vi "MFLI controller -- V1.vi"(6 "pm lorentzian":T1={"Amplitude"=0.011556077084443558, "omega(0)"=1994480.3546612726, "Gamma"=468.65303298958196, "phase"=4.673413347310273, "Q"=4255.771784806969, "Norm  Ampl"=nan, "z (inf)"=2.6527949823343002e-05+0.0007477540585896028i, "4corners"={"z (-pi/2)"=9.277908004825974e-07+0.0007240755403629966i, "z(inf)"=2.6527949823343002e-05+0.0007477540585896028i, "z (pi/2)"=2.8494315967368497e-06+0.0007733542176124632i, "z center"=1.8886111986097237e-06+0.0007487148789877299i, "z(0)"=-2.2750727426123552e-05+0.000749675699385857i, "radius"=2.4658065287076567e-05}} {"z (inf)" format="%#9_9f"; "Q" format="%#9_9f"; "phase" format="%#9_9f"; "Gamma" format="%#9_9f"; "omega(0)" format="%#9_9f"}, 7 "MFLI controller action":T3, 8 "Error In":errorcluster, 9 "sweep parameters":T4={"scan type"=enum."linear", "N"=200, "cursor window"={"left"=2378.60310421286, "right "=2421.6740576496672, "center"=2421.6740576496672, "window"=2421.6740576496672, "cursors"=[], "relative"=0, "absolute"=0, "fixed vertical offset"=2421.6740576496672, "vertical offset"=2421.6740576496672, "skew"=2421.6740576496672, "default window frac"=2421.6740576496672, "kind"=enum."skewed", "skew.left"=2421.6740576496672, "skew.right"=2421.6740576496672, "Plot ref"=refnum, "wing order"=enum."back"}}, 10 "Address":string="DEV3523") -> (0 "Error Out":errorcluster, 1 "Voltage out (V)":cdb[](array[numeric])=[1.7947140397689774e-05+0.0007833320820365352i, 2.4161799481718794e-05+0.000775952788866728i, 1.1398171168621245e-05+0.000786642257900688i, 2.1378172412082557e-05+0.0007803848389655606i, 2.3527732690994892e-05+0.0007832482826747523i, 2.018710709966375e-05+0.000775222845149317i, 2.1052965461761493e-05+0.0007926707916558383i, 2.578223850561299e-05+0.0007823212803731786i, 3.539618410572311e-05+0.000787718994219253i, 2.597151232578711e-05+0.0007817704065018801i, 1.8686171805884874e-05+0.0007845914493356854i, 1.9525315696386483e-05+0.0007805387882637953i, 2.4826921249368033e-05+0.0007881234674194581i, 2.272879706177131e-05+0.0007813422850312608i, 3.06221404697413e-05+0.0007823486263319492i, 2.258400939616162e-05+0.0007913708833571255i, 2.631790122834116e-05+0.0007837787712575242i, 1.877589665213771e-05+0.0007839841799029761i, 2.6429055493472353e-05+0.0007841953035371732i, 2.531443173334934e-05+0.0007816207088595043i, 1.874285359377707e-05+0.0007808713190342089i, 1.3108402421252441e-05+0.0007954138097471226i, 3.648735100939127e-05+0.0007923069644049057i, 1.780208141322794e-05+0.000787914506584111i, 1.0674633557646736e-05+0.0007985997639146586i, 1.546188714204973e-05+0.0007832137363310591i, 2.7415050861775486e-05+0.0007861266083720606i, 1.892095325137887e-05+0.00078571478332542i, 1.7149941209119945e-05+0.0007909710678965998i, 2.3090619534723823e-05+0.0007954700335726445i, 1.4252127066260151e-05+0.0007941394739956062i, 2.5280803103312197e-05+0.0007950770857587566i, 3.212975080358819e-05+0.0007937076512587993i, 1.760575986225483e-05+0.0007908437662837823i, 1.5797629612106515e-05+0.0008016906241041951i, 2.0336565623666577e-05+0.0007986538499861476i, 1.485039288721422e-05+0.000805913067569182i, 2.800021108771304e-05+0.0008038452672883727i, 3.085236077699336e-05+0.0008007500940235448i, 2.129881492750763e-05+0.0008020268042622464i, 3.554295448602157e-06+0.0008061419277043423i, 2.6006880974309018e-05+0.0008047380041059882i, 2.6980288340482813e-05+0.0007933068495095234i, 1.1121641205596253e-05+0.0007879329640180243i, 1.4052702939489842e-05+0.0007929102356114531i, 2.1013801330835356e-05+0.000794124604529898i, 1.626598558143133e-05+0.0007992144555578133i, 1.9885387417361182e-05+0.0008023925593677921i, 2.3694890148735325e-05+0.0007999127658822845i, 8.742127167842653e-06+0.0007970248265530325i, 1.2390541039186939e-05+0.000802933229265029i, 1.483243933116921e-05+0.0007945130842291504i, 9.538450384118407e-06+0.0008015181142112527i, 8.452853567039068e-06+0.0007996583290257916i, 9.257628812788116e-06+0.0008072990894900408i, 1.1681645701650892e-05+0.0008048214754999279i, 6.991344778460933e-06+0.0008067030961880879i, 6.70006580337213e-06+0.0008073005909864577i, 1.3001539764426547e-06+0.0008096541275858048i, 9.044858780017961e-06+0.0008092305338603379i, 6.8739954989232195e-06+0.0008196877992760521i, 1.1866893865625335e-05+0.0008081127484902058i, 1.4235732848233533e-05+0.0008109049546023166i, -7.253909274414909e-07+0.0008132737160652528i, 1.1919072953182212e-06+0.0008099574513290134i, 6.0822942440166985e-06+0.0008105701149382865i, 6.107721292751761e-07+0.0008081147192787912i, -6.260924016914232e-07+0.0008023573773627882i, 1.0163690665722533e-05+0.0008194391328646849i, 4.480674014968536e-06+0.0008205849743930445i, 4.8973529856892366e-06+0.0008076386787247464i, 5.6581191210095015e-06+0.000806127479826389i, -4.4087822711164575e-06+0.0008059624845711934i, 1.4510394587162305e-06+0.0008098497735230208i, -1.1778062880821662e-05+0.000813252261005252i, -1.4585081809649263e-06+0.0008067446723734249i, -2.049438852028277e-06+0.0008100198027864578i, -1.0382074911664064e-05+0.0008125615988908855i, -9.025509273571018e-06+0.000799131903666445i, -2.9031801738195978e-05+0.0008013498166180281i, -1.503670128178013e-05+0.0008049771236715908i, -9.824583841899107e-06+0.0008017113021785598i, -1.8305930062549926e-05+0.000801634818288597i, -8.343519821590533e-06+0.0007944148238707005i, -1.7342980100134644e-05+0.0008019266261863711i, -2.5805486655258495e-05+0.0008042511662542381i, -1.4609085477944594e-05+0.0007968365461772709i, -3.225810668394559e-05+0.0008040385739204086i, -1.5925020670699562e-05+0.0007896679550539058i, -2.9721156155325662e-05+0.0007966369425626446i, -2.5980589283078102e-05+0.0007989693669774635i, -3.771207357449536e-05+0.0008006076206182981i, -2.389227491182575e-05+0.0007991962903134331i, -2.6431435943709224e-05+0.0007911297387391672i, -2.5510202298345777e-05+0.0007948988799588347i, -2.762797414497422e-05+0.0007836354618324298i, -2.673361597360269e-05+0.0007763990308588398i, -3.259733873185462e-05+0.000779768005990542i, -3.222723298379179e-05+0.0007828007824787327i, -2.828513404599954e-05+0.0007775276290306113i, -2.7442523833547298e-05+0.000793928944281358i, -3.3840638588211066e-05+0.0007739791457684968i, -3.521552033589221e-05+0.0007752803450679017i, -3.060214993523709e-05+0.0007727985724455364i, -3.3001774961139156e-05+0.0007626825050958754i, -2.7123296631466546e-05+0.0007718388371642902i, -4.255257124748806e-05+0.0007669934247440899i, -3.38616905459171e-05+0.0007702236915413861i, -1.6438046456581025e-05+0.0007687605220429108i, -2.1381155726845848e-05+0.0007643824005910026i, -2.3810201257203493e-05+0.0007613015392465492i, -1.9462442471918776e-05+0.0007633144454623645i, -1.3585483527818204e-05+0.0007618983596237723i, -1.0020322802721557e-05+0.0007542783314976581i, -1.6568035020492665e-05+0.0007604883692166231i, -2.298965314341451e-05+0.0007605745114614172i, -1.426624995789593e-05+0.0007620358437436652i, -2.0535935486666456e-05+0.0007556581560188897i, -1.7212791773991207e-05+0.0007694160367379733i, -1.3989350285665814e-05+0.0007610824084265354i, -1.400786973531673e-05+0.0007577904317961574i, -1.8543965545354192e-05+0.0007530162033055729i, -9.895804742435434e-06+0.0007541670555862725i, -1.182271182669738e-05+0.0007564713874682483i, -1.3404755357029001e-06+0.0007534417952496631i, -2.540462766068613e-07+0.0007474275871299063i, -1.3033629927126234e-05+0.0007444921079673166i, -3.0160083868227686e-06+0.0007582129479981829i, -4.11029992957941e-06+0.0007583807524470322i, 7.493713398352082e-07+0.0007579380829191913i, 2.5281812647964257e-06+0.0007541958762077274i, 8.73539368986802e-06+0.0007522473143012331i, 1.9213280530955755e-06+0.0007605324767174049i, 1.203060825731675e-05+0.0007498036420013713i, 1.0818751572551014e-05+0.0007547940269417837i, -4.571233688458752e-07+0.0007544590167344752i, 9.230090843752823e-06+0.0007623847234129125i, 7.672275192460286e-06+0.0007716896457850033i, 3.724034311421603e-06+0.0007561014117147125i, 9.7155864125662e-06+0.0007589951489191279i, 1.9036995429984916e-05+0.0007591741692719116i, 2.993680932359062e-06+0.0007534712712104994i, 1.3241246094315913e-05+0.0007587625553173011i, -2.3831181061984005e-06+0.0007575792067900815i, 1.2540396106127523e-05+0.0007558400475810648i, 1.543095500398932e-05+0.000755777378292965i, 1.1838465016666725e-05+0.0007658480220963351i, 9.470274217777834e-06+0.0007540965860302497i, 1.1865047704820388e-06+0.0007644510764610753i, 8.466614501436925e-06+0.0007562911083152517i, 1.9635644675163006e-05+0.0007559176668360705i, 1.5652852679989877e-05+0.0007649946688499482i, 1.6426636753466735e-05+0.0007582663668041872i, 1.783993128756037e-05+0.0007500404991851605i, 1.0973498727102639e-05+0.0007677684950478176i, 6.5668631545965845e-06+0.0007641153292205771i, 1.3746500234922546e-05+0.0007664765390748459i, 1.313554086582413e-05+0.0007479720215016787i, 1.625381320400517e-05+0.0007647049671020328i, 2.2693736106716893e-05+0.0007611466185671932i, 1.063844260429601e-05+0.0007676103000567756i, 8.724583869754299e-06+0.000760347093192157i, 2.9722842506345163e-05+0.0007540097204672849i, 1.6862222772198565e-05+0.000766293135282761i, 1.3051362850258507e-05+0.0007733673736354523i, 2.2415757122129878e-05+0.0007654096173430668i, 1.9622996446211543e-05+0.0007736139273376037i, 1.683381240870021e-05+0.000769355971514549i, 2.4967869902296118e-05+0.0007724409640612171i, 2.8596211545327962e-05+0.0007752939199550868i, 2.225968676640701e-05+0.0007710920251662428i, 2.1970411972993085e-05+0.0007627460700343397i, 2.5802859334681428e-05+0.0007671525469896707i, 2.615942835909015e-05+0.0007751067057729683i, 1.8932634273345313e-05+0.0007677137578110834i, 2.1265462386763993e-05+0.0007613570302130178i, 2.3909834310153683e-05+0.0007645137904720627i, 2.132736423011049e-05+0.0007730512507980843i, 2.1087956052805902e-05+0.0007702563958984105i, 2.764070526034425e-05+0.0007666090142313147i, 2.8825530239163648e-05+0.0007725496436598947i, 1.729867104820557e-05+0.0007754645204788762i, 2.487072463451332e-05+0.0007644461527692902i, 3.0526769806143105e-05+0.0007779116078184439i, 2.287845117386975e-05+0.0007798770845173779i, 2.062062215054171e-05+0.0007695059261644529i, 3.166101379526004e-05+0.0007710586797811611i, 3.2229803655377746e-05+0.0007608600021022252i, 1.7318390860162808e-05+0.000778979904629944i, 2.77694380055688e-05+0.0007824131662293659i, 1.618981594429285e-05+0.0007837812626205225i, 1.969374805457943e-05+0.0007784960435336005i, 2.6395515116600305e-05+0.0007839889300699569i, 1.9374879828210753e-05+0.0007738837953792744i, 2.6467750332230046e-05+0.0007704428527729637i, 2.345675627557808e-05+0.0007902514134248894i, 1.947387304571401e-05+0.0007802039945152633i, 2.3576121662894066e-05+0.000779339309085434i, 1.2183886115930586e-05+0.0007743616063633677i, 2.839087087866531e-05+0.0007817038850823851i], 2 "sweep time":dbl=5.15086802226142, 3 "Freq out (Hz)":dbl[](array[numeric])=[1966839.6309110236, 1980604.250263973, 1985224.7472832582, 1987541.939474813, 1988935.024090971, 1989865.2790140666, 1990530.774699402, 1991030.6713716055, 1991420.1075499407, 1991732.1886906968, 1991987.9930281865, 1992201.5787029702, 1992382.681702111, 1992538.2583730097, 1992673.4113469622, 1992791.9684604905, 1992896.857472874, 1992990.3559479269, 1993074.26226771, 1993150.01536806, 1993218.7802804522, 1993281.510355006, 1993338.993258559, 1993391.8854780952, 1993440.7385467284, 1993486.019219916, 1993528.1251697806, 1993567.3973176058, 1993604.1296157013, 1993638.5768735865, 1993670.9610699513, 1993701.47648153, 1993730.2938797704, 1993757.5639871648, 1993783.4203412689, 1993807.9816815516, 1993831.3539493254, 1993853.6319720135, 1993874.9008884, 1993895.237360179, 1993914.7106062812, 1993933.3832895095, 1993951.3122795206, 1993968.5493118234, 1993985.1415589666, 1994001.1321272748, 1994016.5604902243, 1994031.4628676944, 1994045.8725588291, 1994059.8202350016, 1994073.3341983613, 1994086.4406105939, 1994099.1636958327, 1994111.5259210719, 1994123.5481569448, 1994135.2498213276, 1994146.6490078745, 1994157.7626013076, 1994168.606381035, 1994179.1951144587, 1994189.5426411608, 1994199.6619489975, 1994209.5652430046, 1994219.2640079013, 1994228.769064887, 1994238.0906233364, 1994247.238327932, 1994256.2213017046, 1994265.0481854002, 1994273.7271735466, 1994282.2660475457, 1994290.6722060877, 1994298.9526931448, 1994307.1142237792, 1994315.163207975, 1994323.1057726797, 1994330.9477822206, 1994338.6948572523, 1994346.3523923666, 1994353.925572489, 1994361.419388173, 1994368.8386498927, 1994376.1880014255, 1994383.4719324044, 1994390.694790122, 1994397.8607906487, 1994404.974029333, 1994412.0384907408, 1994419.058058085, 1994426.036522199, 1994432.9775900966, 1994439.8848931633, 1994446.761995016, 1994453.61239907, 1994460.439555851, 1994467.246870078, 1994474.0377075572, 1994480.8154019113, 1994487.583261174, 1994494.3445742792, 1994501.1026174715, 1994507.8606606638, 1994514.621973769, 1994521.3898330317, 1994528.1675273858, 1994534.958364865, 1994541.765679092, 1994548.592835873, 1994555.443239927, 1994562.3203417796, 1994569.2276448463, 1994576.168712744, 1994583.147176858, 1994590.1667442021, 1994597.2312056099, 1994604.3444442942, 1994611.5104448209, 1994618.7333025385, 1994626.0172335175, 1994633.3665850502, 1994640.78584677, 1994648.279662454, 1994655.8528425763, 1994663.5103776907, 1994671.2574527224, 1994679.0994622633, 1994687.042026968, 1994695.0910111638, 1994703.2525417982, 1994711.5330288552, 1994719.9391873972, 1994728.4780613964, 1994737.1570495428, 1994745.9839332383, 1994754.9669070109, 1994764.1146116066, 1994773.436170056, 1994782.9412270417, 1994792.6399919384, 1994802.5432859454, 1994812.6625937822, 1994823.0101204843, 1994833.598853908, 1994844.4426336354, 1994855.5562270684, 1994866.9554136153, 1994878.6570779982, 1994890.679313871, 1994903.0415391102, 1994915.764624349, 1994928.8710365817, 1994942.3849999413, 1994956.3326761138, 1994970.7423672485, 1994985.6447447187, 1995001.0731076682, 1995017.0636759764, 1995033.6559231195, 1995050.8929554224, 1995068.8219454335, 1995087.4946286618, 1995106.967874764, 1995127.304346543, 1995148.5732629295, 1995170.8512856176, 1995194.2235533914, 1995218.784893674, 1995244.6412477782, 1995271.9113551725, 1995300.728753413, 1995331.2441649917, 1995363.6283613564, 1995398.0756192417, 1995434.8079173372, 1995474.0800651624, 1995516.1860150269, 1995561.4666882146, 1995610.3197568478, 1995663.211976384, 1995720.694879937, 1995783.4249544907, 1995852.189866883, 1995927.942967233, 1996011.849287016, 1996105.347762069, 1996210.2367744525, 1996328.7938879807, 1996463.9468619332, 1996619.523532832, 1996800.6265319728, 1997014.2122067565, 1997270.016544246, 1997582.0976850023, 1997971.5338633375, 1998471.430535541, 1999136.9262208764, 2000067.1811439719, 2001460.26576013, 2003777.4579516847, 2008397.95497097])   [LabVIEW 2016]
uses:
  <instrlib>/Zurich Instruments LabOne/Zurich Instruments LabOne.lvlib
  MFLI controller action.ctl
  cursor winow.ctl
  sweep parameters.ctl
  circle corners.ctl
  lorentzian.ctl
panel:
  out "Thermometer":i32(slide) scale=0.0..100.0
  out "Selected Device":string="DEV3523"
  out "ind":i64=-1
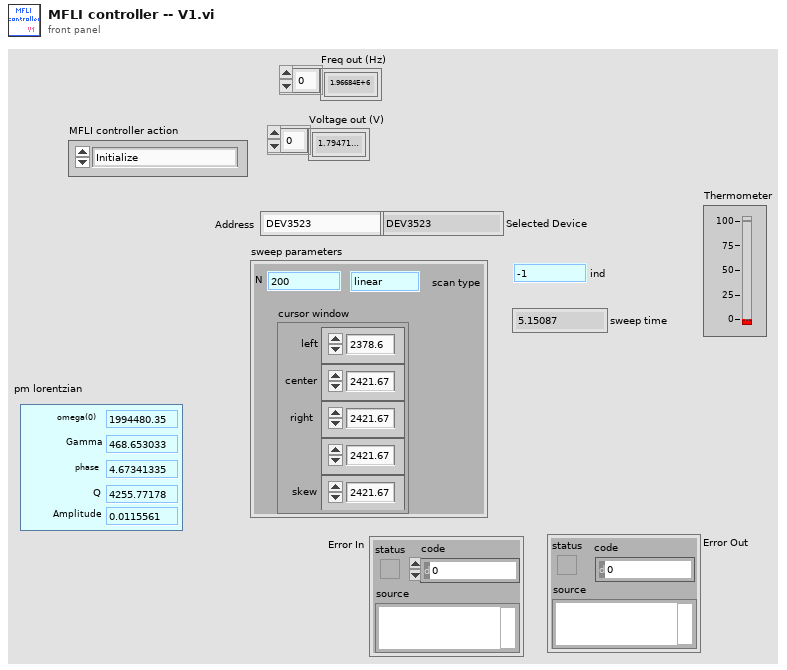
[diagram p1: front panel]
types:
  T1 = typedef "lorentzian.ctl" = cluster{"Amplitude":dbl, "omega(0)":dbl, "Gamma":dbl, "phase":dbl, "Q":dbl, "Norm  Ampl":dbl, "z (inf)":cdb, "4corners":T2}
  T2 = typedef "circle corners.ctl" = cluster{"z (-pi/2)":cdb, "z(inf)":cdb, "z (pi/2)":cdb, "z center":cdb, "z(0)":cdb, "radius":dbl}
  T3 = typedef "MFLI controller action.ctl" = enum16{"Initialize", "Scan frequency", "open", "close", "read", "circle PLL"}
  T4 = typedef "sweep parameters.ctl" = cluster{"scan type":enum16{"linear", "arctan"}, "N":i64, "cursor window":T5}
  T5 = typedef "cursor winow.ctl" = cluster{"left":dbl, "right ":dbl, "center":dbl, "window":dbl, "cursors":i32[], "relative":i32, "absolute":i32, "fixed vertical offset":dbl, "vertical offset":dbl, "skew":dbl, "default window frac":dbl, "kind":enum16{"symmetric", "skewed", "fancy"}, "skew.left":dbl, "skew.right":dbl, "Plot ref":refnum<vi>, "wing order":enum16{"forw", "back"}}
  T6 = typedef "Zurich Instruments LabOne.lvlib/ziTypeHandle.ctl" = cluster{"handleValid":bool, "Conn":u64, "Path Prefix":string, "Handle":u64, "Connected":bool, "Clockbase(s)":dbl}
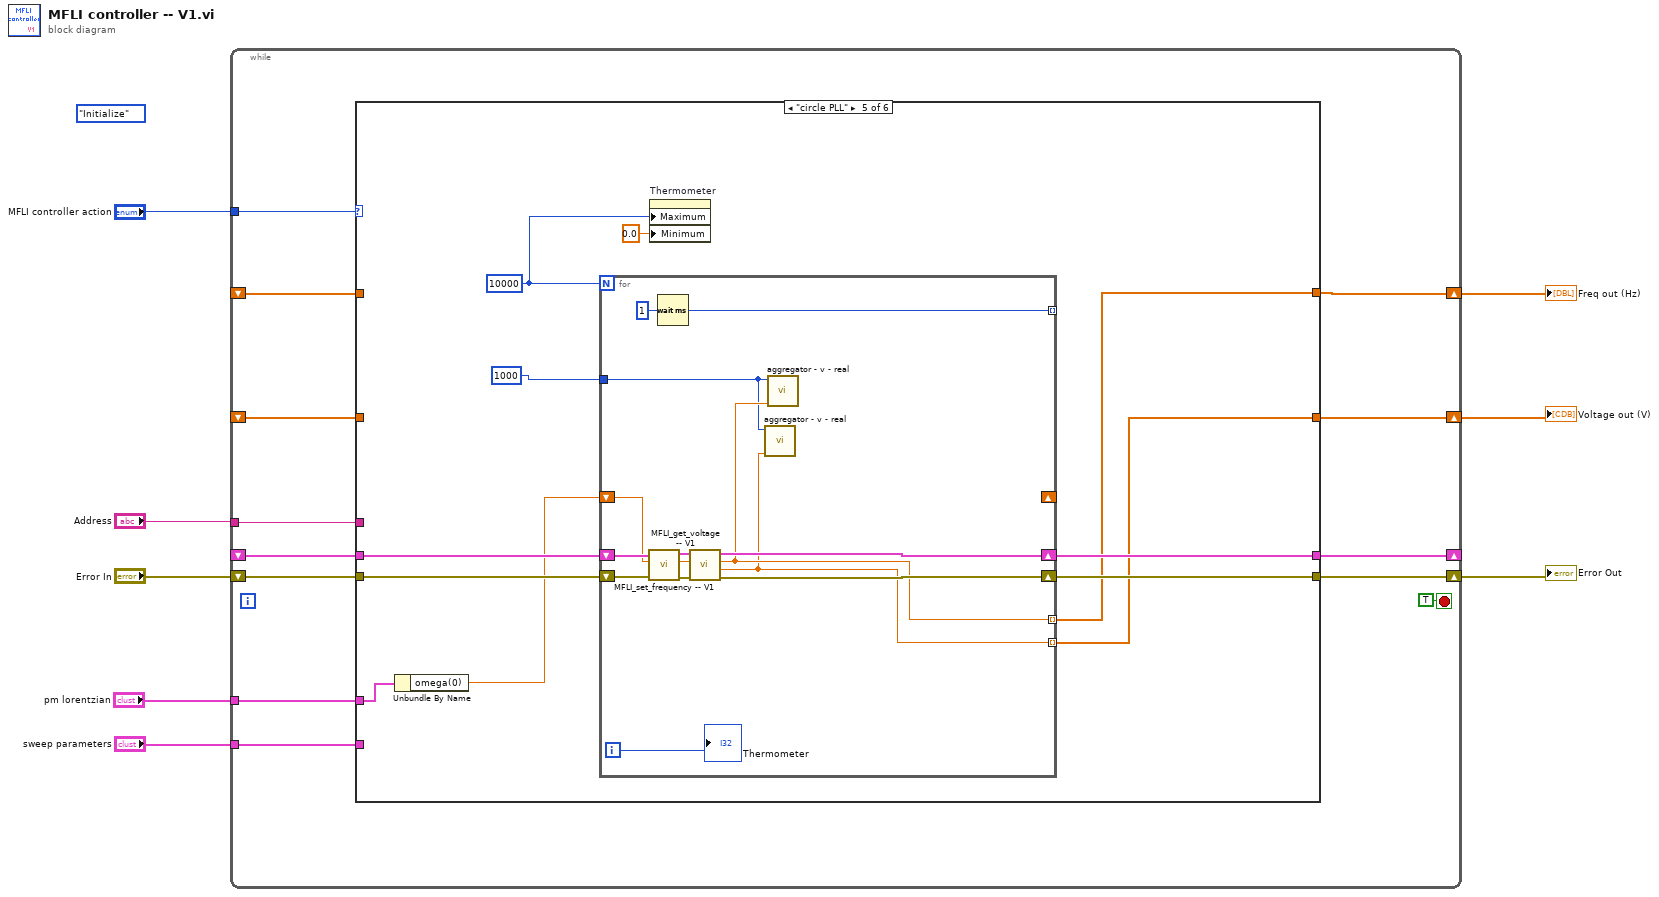
[diagram p0: block diagram]
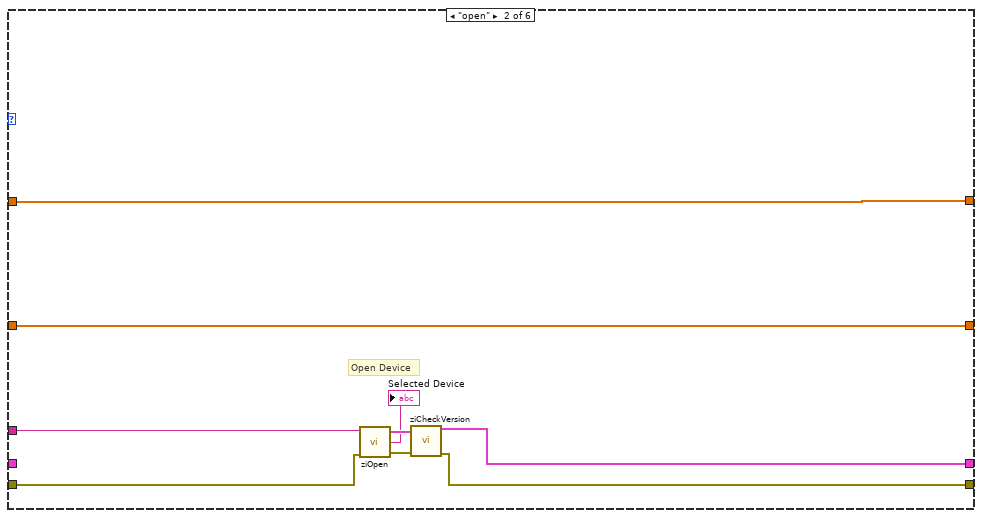
[diagram p3: hidden frame]
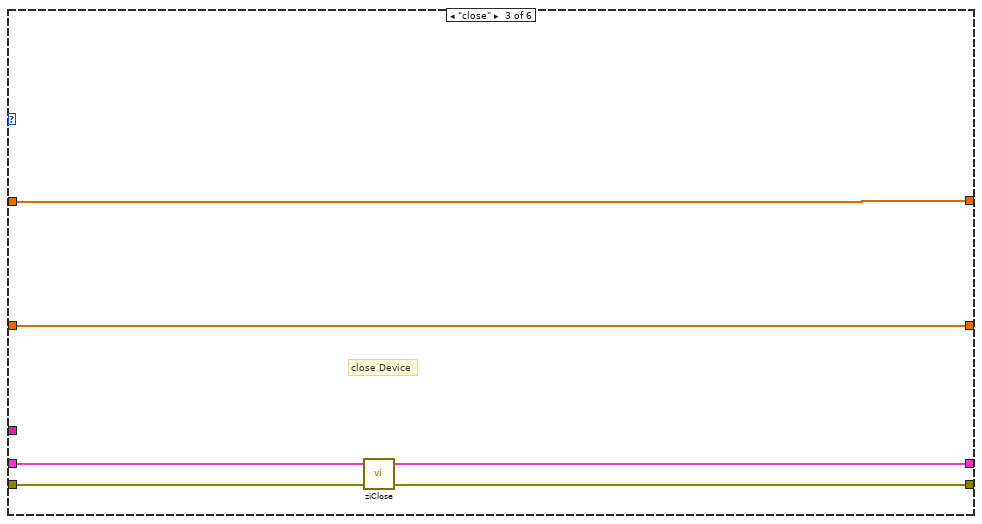
[diagram p4: hidden frame]
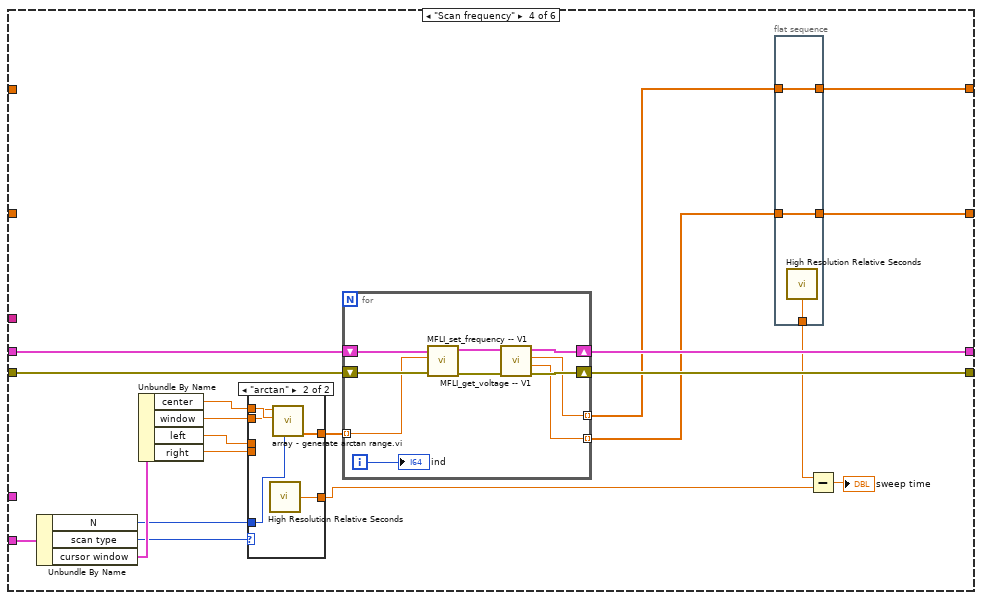
[diagram p5: hidden frame]
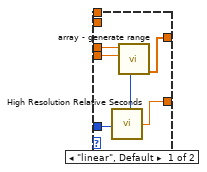
[diagram p6: hidden frame]
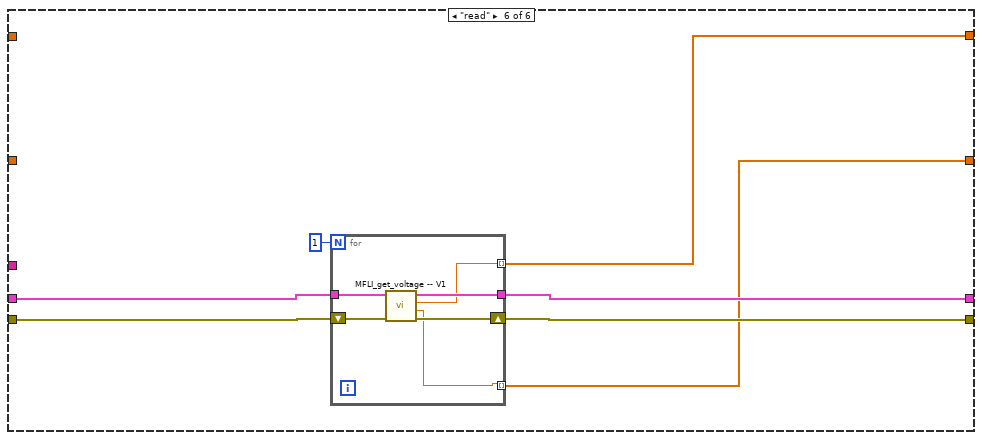
[diagram p7: hidden frame]
diagram:
  (unwired) MFLI_controller_action."Initialize" ("MFLI controller action")
  n1 = while {
    shift-right: [w21] -> w8
    shift-left: _ -> [w19]
    shift-right: [w20] -> w7
    shift-left: _ -> [w18]
    shift-right: [w15] -> _
    shift-left: _ -> [w16]
    shift-right: [w13] -> w2
    shift-left: "Error In" -> [w14]
    tunnel: "MFLI controller action" -> [w12]
    tunnel: "sweep parameters" -> [w11]
    tunnel: "Address" -> [w10]
    tunnel: "pm lorentzian" -> [w9]
    stop <- TRUE stop-if-true
    n2 = case shown="\"circle PLL\"" w12 {
      tunnel: [w25 w34 w40 w60 w89 w109] -> w21
      tunnel: [w24 w33 w39 w59 w90 w110] -> w20
      tunnel: w19 -> [w25 w34 w40 _ _ _]
      tunnel: w18 -> [w24 w33 w39 _ _ _]
      tunnel: w16 -> [w23 _ w35 w57 w94 w115]
      tunnel: [w23 w26 w36 w56 w93 w114] -> w15
      tunnel: w14 -> [w22 w28 w38 w55 w92 w113]
      tunnel: [w22 w27 w37 w54 w91 w112] -> w13
      tunnel: w11 -> [_ _ _ w44 _ _]
      tunnel: w10 -> [_ w29 _ _ _ _]
      tunnel: w9 -> [_ _ _ _ w87 _]
      frame "Initialize", Default {
      }
      frame "open" {
        # "Open Device"
        n3 = call "ziOpen.vi"("Error In"=w28, "Address"=w29) -> ("Error Out"=w32:errorcluster, "Selected Device"=→"Selected Device":string, "HandleOut"=w31:T6)  [unwired: 2 out]
        n4 = call <instrlib>:"ziCheckVersion.vi"("Handle In"=w31, "Error In"=w32) -> ("Handle Out"=w26:T6, "Error Out"=w27:errorcluster)  [unwired: 12 in]
      }
      frame "close" {
        # "close Device"
        n5 = call "ziClose.vi"("Error In"=w38, "Handle In"=w35) -> ("Error Out"=w37:errorcluster, "Handle Out"=w36:T6)  [unwired: 2 in]
      }
      frame "Scan frequency" {
        n6 = Unbundle By Name(w44) -> ("N"=w42:i64, "scan type"=w41:enum16{"linear", "arctan"}, "cursor window"=w43:T5)
        n7 = Unbundle By Name(w43) -> ("center"=w51:dbl, "window"=w50:dbl, "left"=w49:dbl, "right"=w48:dbl)
        n8 = case shown="\"arctan\"" w41 {
          tunnel: [w65 w70] -> w58
          tunnel: w51 -> [_ w69]
          tunnel: w50 -> [_ w68]
          tunnel: w49 -> [w64 _]
          tunnel: w48 -> [w63 _]
          tunnel: [w62 w67] -> w47
          tunnel: w42 -> [w61 w66]
          frame "linear", Default {
            n9 = call <vilib>:"High Resolution Relative Seconds.vi"() -> ("relative seconds"=w62:dbl)
            n10 = call "array - generate range.vi"("N"=w61, "freq max"=w63, "freq min"=w64) -> ("Array"=w65:dbl[])  [unwired: 7 in, 1 out]
          }
          frame "arctan" {
            n11 = call <vilib>:"High Resolution Relative Seconds.vi"() -> ("relative seconds"=w67:dbl)
            n12 = call "array - generate arctan range.vi.vi"("N"=w66, "omega0"=w69, "gamma"=w68) -> ("Array"=w70:dbl[])  [unwired: 8 in]
          }
        }
        n13 = for {
          shift-right: [w79] -> w56
          shift-left: w57 -> [w75]
          shift-right: [w80] -> w54
          shift-left: w55 -> [w73]
          tunnel: w58 -> [w71] mode=indexing
          tunnel: [w77] -> w53 mode=indexing
          tunnel: [w78] -> w52 mode=indexing
          i -> [w76]
          n14 = call "MFLI_set_frequency -- V1.vi"("Error In"=w73, "Freq in (Hz)"=w71, "Handle In"=w75) -> ("Error Out"=w72:errorcluster, "Handle Out"=w74:T6)  [unwired: 5 in, 2 out]
          n15 = call "MFLI_get_voltage -- V1.vi"("Error In"=w72, "Handle In"=w74) -> ("Error Out"=w80:errorcluster, "z out (V)"=w78:cdb, "Freq out (Hz)"=w77:dbl, "Handle Out"=w79:T6)  [unwired: 6 in]
          "ind" <- w76
        }
        n16 = flat-sequence {
          tunnel: w53 -> [w83]
          tunnel: [w83] -> w60
          tunnel: w52 -> [w82]
          tunnel: [w82] -> w59
          tunnel: [w81] -> w46
          frame #0 {
            n17 = call <vilib>:"High Resolution Relative Seconds.vi"() -> ("relative seconds"=w81:dbl)
          }
        }
        n18 = Subtract(x=w46, y=w47) -> (x-y=→"sweep time":dbl)
      }
      frame "circle PLL" {
        w85 = 10000
        n19 = Unbundle By Name(w87) -> ("omega(0)"=w86:dbl)
        n20 = for {
          N: w85 -> [_]
          shift-right: [w107] -> w93
          shift-left: w94 -> [w106]
          shift-right: [w108] -> w91
          shift-left: w92 -> [w104]
          tunnel: [w97] -> w89 mode=indexing
          tunnel: [w96] -> w90 mode=indexing
          tunnel: [w100] -> _ mode=indexing
          tunnel: 1000 -> [w95]
          shift-right: _ -> [_]
          shift-left: w86 -> [w98]
          i -> [w102]
          n21 = call "MFLI_set_frequency -- V1.vi"("Error In"=w104, "Freq in (Hz)"=w98, "Handle In"=w106) -> ("Error Out"=w103:errorcluster, "Freq out (Hz)"=w99:dbl, "Handle Out"=w105:T6)  [unwired: 5 in, 1 out]
          n22 = Wait (ms)(milliseconds to wait=u32 1) -> (millisecond timer value=w100:u32)
          n23 = call "MFLI_get_voltage -- V1.vi"("Error In"=w103, "Freq in (Hz)"=w99, "Handle In"=w105) -> ("Error Out"=w108:errorcluster, "z out (V)"=w96:cdb, "Freq out (Hz)"=w97:dbl, "Handle Out"=w107:T6)  [unwired: 5 in]
          n24 = call "aggregator - v - real.vi"("number"=w96, "requested size"=w95) -> ()  [unwired: 7 in, 3 out]
          n25 = call "aggregator - v - real.vi"("number"=w97, "requested size"=w95) -> ()  [unwired: 7 in, 3 out]
          "Thermometer" <- w102
        }
        n26 = property on="Thermometer" class="Slide (strict)"("Maximum"=w85, "Minimum"=0.0 ("Data Entry Limits:Minimum")) -> ()  [unwired: 2 in, 2 out]
      }
      frame "read" {
        n27 = for {
          N: 1 -> [_]
          tunnel: w115 -> [w121]
          tunnel: [w120] -> w114
          shift-right: [w118] -> w112
          shift-left: w113 -> [w119]
          tunnel: [w117] -> w109 mode=indexing
          tunnel: [w116] -> w110 mode=indexing
          n28 = call "MFLI_get_voltage -- V1.vi"("Error In"=w119, "Handle In"=w121) -> ("Error Out"=w118:errorcluster, "z out (V)"=w116:cdb, "Freq out (Hz)"=w117:dbl, "Handle Out"=w120:T6)  [unwired: 6 in]
        }
      }
    }
  }
  "Error Out" <- w2
  "Freq out (Hz)" <- w8
  "Voltage out (V)" <- w7
